vi "SineWaveGraph(ForLoop).vi"() -> ()   [LabVIEW 2015]
panel:
  out "Waveform Graph":cluster{"y":dbl, "y":dbl, dbl[]}(graph)
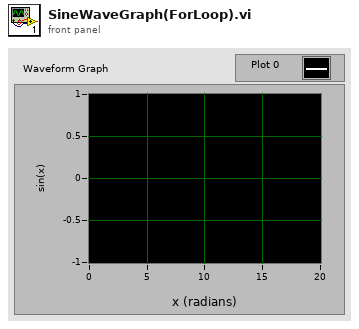
[diagram p1: front panel]
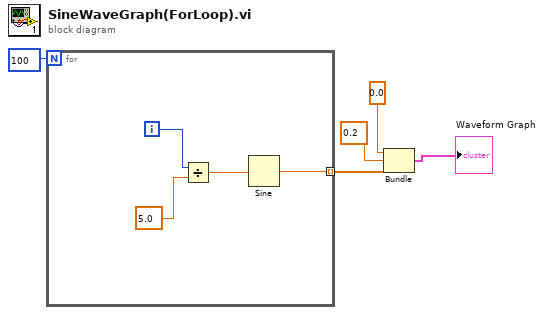
[diagram p0: block diagram]
diagram:
  n1 = for {
    N: 100 -> [_]
    tunnel: [w7] -> w4 mode=indexing
    i -> [w8]
    n2 = Divide(x=w8, y=5.0) -> (x/y=w6:dbl)
    n3 = Sine(x=w6) -> (sin(x)=w7:dbl)
  }
  n4 = Bundle("y"=0.0, "y"=0.2, w4) -> (→"Waveform Graph":cluster{"y":dbl, "y":dbl, dbl[]})  [unwired: 1 in]
